vi "colorarraytopixmap.vi"(11 "Colors":u32[](array[colorbox])) -> (3 "output cluster":T1)   [LabVIEW 2020, in "3DPC_SurfacePlot.xctl"]
uses:
  <vilib>/Native 3D Graph/xcontrol/3DPC_SurfacePlot.xctl
  <vilib>/picture/picture.llb/imagedata.ctl
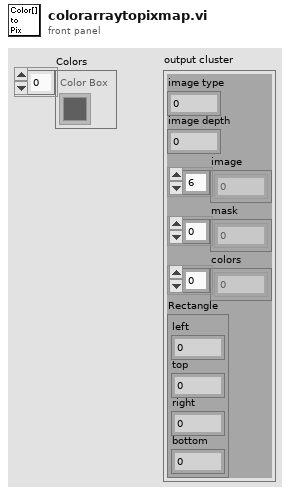
[diagram p1: front panel]
types:
  T1 = typedef "imagedata.ctl" = cluster{"image type":i32, "image depth":i32, "image":u8[], "mask":u8[], "colors":u32[], "Rectangle":cluster{"left":i16, "top":i16, "right":i16, "bottom":i16}}
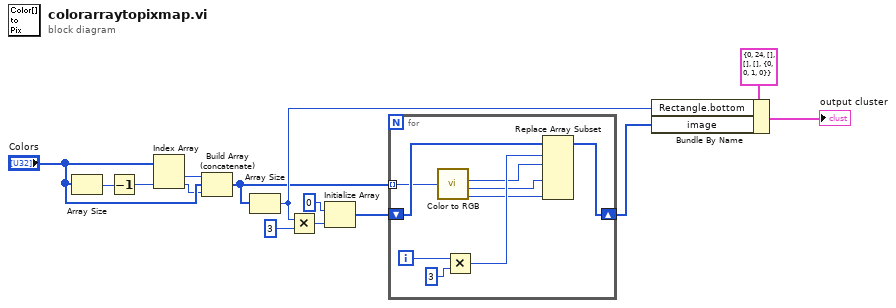
[diagram p0: block diagram]
diagram:
  n1 = Array Size(array="Colors") -> (size(s)=w6:i32)
  n2 = Decrement(x=w6) -> (x-1=w2:i32)
  n3 = Index Array(array="Colors", index #2=w2) -> (element #1=w5:u32, element #2=w1:u32)  [unwired: 1 in]
  n4 = Build Array (concatenate)(w5, "Colors", w1) -> (w3:u32[])
  n5 = Array Size(array=w3) -> (size(s)=w7:i32)
  n6 = Multiply(x=w7, y=3 ("element")) -> (x*y=w11:i32)
  n7 = Initialize Array(u8 0 ("element"), w11) -> (w10:u8[])
  n8 = for {
    shift-right: [w16] -> w9
    shift-left: w10 -> [w23]
    tunnel: w3 -> [w15] mode=indexing
    i -> [w22]
    n9 = call <vilib>:"Color to RGB.vi"("Color"=w15) -> ("R"=w17:u8, "G"=w18:u8, "B"=w19:u8)  [unwired: 1 out]
    n10 = Multiply(x=w22, y=3) -> (x*y=w20:i32)
    n11 = Replace Array Subset(array=w23, new element #1=w17, index #1=w20, new element #2=w18, new element #3=w19) -> (w16:u8[])  [unwired: 2 in]
  }
  n12 = Bundle By Name(cluster=T1 {"image type"=0, "image depth"=24, "image"=[], "mask"=[], "colors"=[], "Rectangle"={"left"=0, "top"=0, "right"=1, "bottom"=0}} ("image data"), "Rectangle.bottom"=w7, "image"=w9) -> (→"output cluster":T1)
